vi "Set_Remote_Local_XDM3051.vi"(8 "error in":errorcluster, 10 "REM_LOCAL":enum16{""}(ring), 11 "RS232_Input":refnum<visa-resource-name>) -> (0 "error out":errorcluster, 2 "response":string, 3 "RS232_Output":refnum<visa-resource-name>)   [LabVIEW 2017]
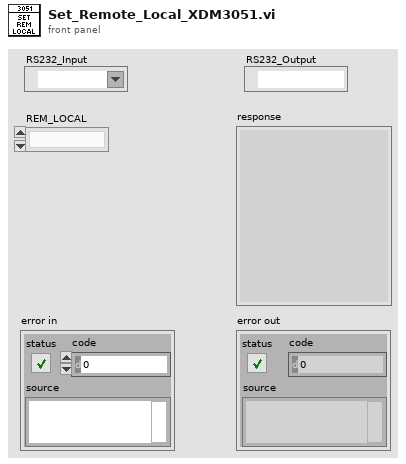
[diagram p1: front panel]
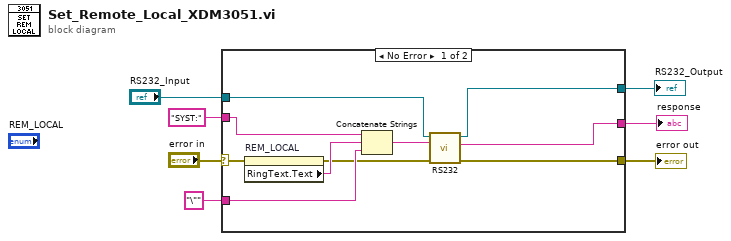
[diagram p0: block diagram]
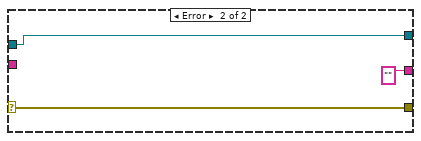
[diagram p2: hidden frame]
diagram:
  n1 = case shown="No Error" "error in" {
    selector: "error in" -> [w9 w20]
    tunnel: [w17 w20] -> w6
    tunnel: "RS232_Input" -> [w16 w19]
    tunnel: "SYST:" ("command") -> [w13 _]
    tunnel: [w15 "" ("response")] -> w3
    tunnel: [w14 w19] -> w2
    tunnel: "\"" ("command") -> [w12 _]
    frame No Error {
      n2 = property on="REM_LOCAL" class="Enum (strict)"(error in=w9) -> (error out=w8:errorcluster, "RingText.Text"=w10:string)  [unwired: 1 in, 1 out]
      n3 = Concatenate Strings(w13, w10, w12) -> (w11:string)
      n4 = call "RS232.vi"("error in"=w8, "command"=w11, "RS232_Input"=w16) -> ("error out"=w17:errorcluster, "response"=w15:string, "RS232_Output"=w14:refnum<visa-resource-name>)  [unwired: 6 in]
    }
    frame Error {
    }
  }
  "error out" <- w6
  "RS232_Output" <- w2
  "response" <- w3
